vi "Get SOC OCV Curve.vi"(0 "reference in":refnum<class "Battery.lvclass">, 5 "Error In":errorcluster) -> (14 "reference out":refnum<class "Battery.lvclass">, 16 "SOC OCV Curve":dbl[][](array[numeric]), 19 "Error Out":errorcluster)   [LabVIEW 2023, in "Battery.lvclass"]
uses:
  Battery.lvclass
panel:
  out "return value":string
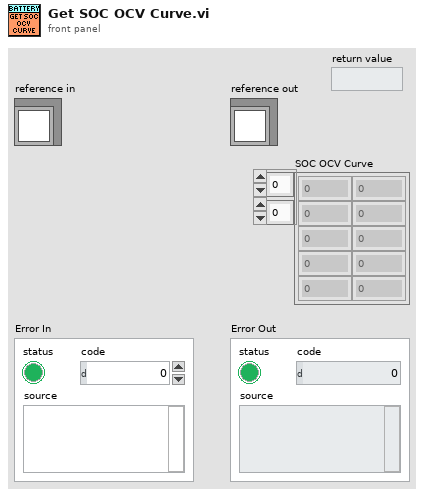
[diagram p1: front panel]
types:
  T1 = typedef "Battery.lvclass/ObjectAttributes.ctl" = cluster{"Python module":path, "Python Session":refnum<k35>, "PybammWrapper":refnum<k38>, "simulation loaded":bool, "simulation enabled":bool, "SOC OCV Curve":dbl[][], "Open Circuit Voltage (V)":dbl, "Terminal Voltage (V)":dbl, "State of Charge (%)":dbl, "# Cells in Series":u16, "# Cells in Parallel":u16, "Simulation Parameters":T2, "Power Module":refnum<class "PowerModuleInterface.lvclass">}
  T2 = typedef "Battery.lvclass/Simulation Parameters.ctl" = cluster{"num_rc_pairs":i32, "R0":dbl, "R1":dbl, "C1":dbl, "R2":dbl, "C2":dbl, " nominal_capacity_Ah":dbl, "upper_voltage_cutoff":dbl, "lower_voltage_cutoff":dbl}
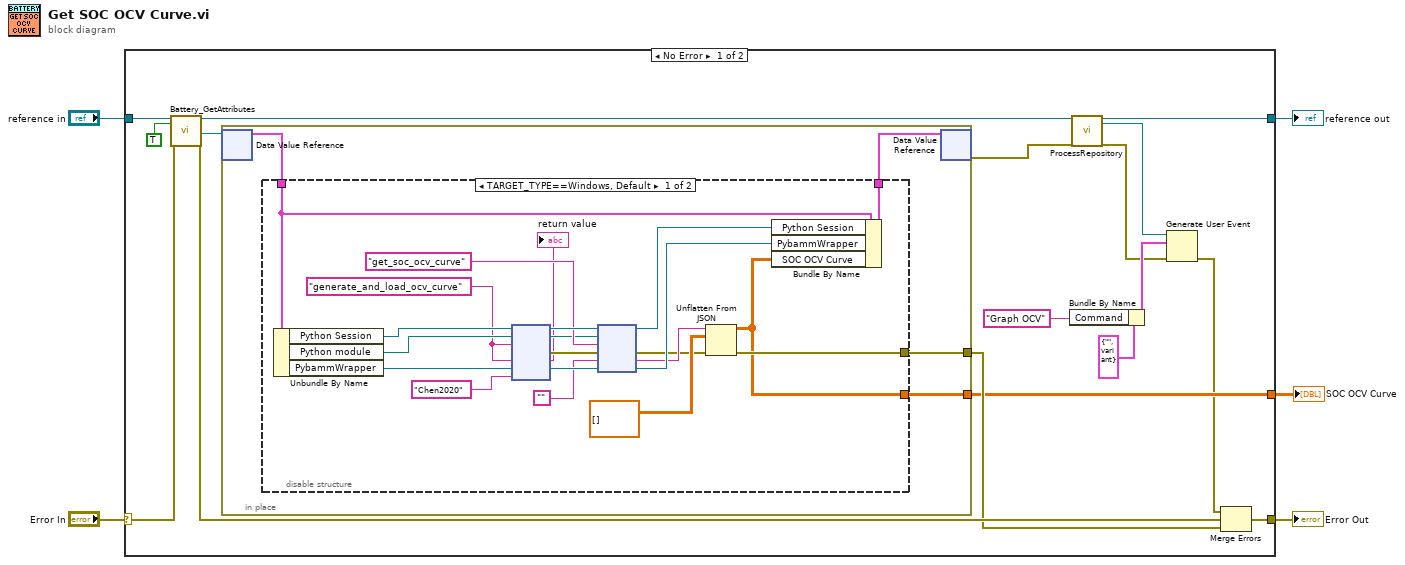
[diagram p0: block diagram]
diagram:
  n1 = case shown="No Error" "Error In" {
    selector: "Error In" -> [w22 w49]
    tunnel: [w21 w49] -> w4
    tunnel: [w8 w48] -> w2
    tunnel: "reference in" -> [w15 w48]
    tunnel: [w16 _] -> w1
    frame No Error {
      n2 = call "Battery_GetAttributes.vi"("reference in"=w15, "OnlyGetDvrReference(False)"=TRUE, "Error In"=w22) -> ("reference out"=w9:refnum<class "Battery.lvclass">, "DataRef"=w20:refnum<data-value>, "Error Out"=w18:errorcluster)  [unwired: 13 in, 1 out]
      n3 = in-place {
        in-place-border: [w24] -> w17
        in-place-border: [w23] -> w16
        n4 = in-place-dvr #1(w20) -> (w25:T1)  [unwired: 1 out]
        n5 = disable-structure shown="TARGET_TYPE==Windows, Default" {
          disable-tunnel: [w46 w47] -> w26
          disable-tunnel: w25 -> [w45 w47]
          disable-tunnel: [w42 _] -> w24
          disable-tunnel: [w41 _] -> w23
          frame condition #0 (active) {
            w28 = "generate_and_load_ocv_curve" ("function name")
            n6 = Unbundle By Name(w45) -> ("Python Session"=w43:refnum<k35>, "Python module"=w31:path, "PybammWrapper"=w44:refnum<k38>)
            n7 = node(w43, w31, w28, w28, w44, "Chen2020" ("function name")) -> (w39:refnum<k35>, w30:errorcluster, →"return value":string, w38:refnum<k38>)  [unwired: 2 in, 2 out]
            n8 = node(w39, w31, "get_soc_ocv_curve" ("function name"), w30, "", w38) -> (w36:refnum<k35>, w29:errorcluster, w32:string, w37:refnum<k38>)  [unwired: 2 out]
            n9 = Unflatten From JSON(JSON string=w32, type and defaults=dbl[][] [], error in (no error)=w29) -> (value=w41:dbl[][], error out=w42:errorcluster)  [unwired: 4 in]
            n10 = Bundle By Name(cluster=w45, "Python Session"=w36, "PybammWrapper"=w37, "SOC OCV Curve"=w41) -> (w46:T1)
          }
          frame condition #1 {
          }
        }
        n11 = in-place-dvr #1(w26) -> (w6:errorcluster)  [unwired: 1 out]
      }
      n12 = Bundle By Name(cluster=cluster{"Command":string, "Data":variant} {"Command"="", "Data"=variant} ("MessageToProcess"), "Command"="Graph OCV") -> (w14:cluster{"Command":string, "Data":variant})
      n13 = call "ProcessRepository.vi"("reference in"=w9, "Error In"=w6) -> ("reference out"=w8:refnum<class "Battery.lvclass">, "EventsToProcess"=w12:refnum<user-event>, "Error Out"=w13:errorcluster)  [unwired: 10 in, 5 out]
      n14 = Generate User Event(user event=w12, event data cluster=w14, error in=w13) -> (error out=w7:errorcluster)  [unwired: 1 in, 1 out]
      n15 = Merge Errors(w7, w18, w17) -> (w21:errorcluster)
    }
    frame Error {
    }
  }
  "Error Out" <- w4
  "reference out" <- w2
  "SOC OCV Curve" <- w1
